vi "RAMP_uptade_scan_steps_indicators.vi"(4 "Total # steps":i32, 5 "error in":errorcluster) -> (6 "slider":u8, 7 "scan step":i32, 8 "error out":errorcluster)   [LabVIEW 2015]
uses:
  GLOBAL/Global_MAIN.vi
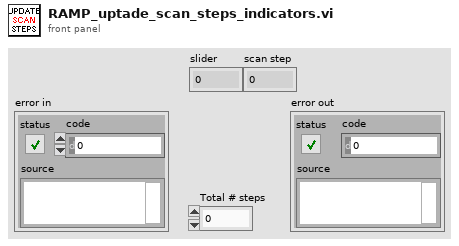
[diagram p1: front panel]
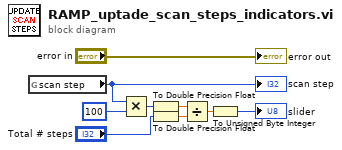
[diagram p0: block diagram]
diagram:
  n1 = global read "Global_MAIN.vi" "scan step"() -> (w6:i32)
  "scan step" <- w6
  n2 = Multiply(x=w6, y=100) -> (x*y=w8:i32)
  n3 = To Double Precision Float(number=w8) -> (double precision float=w2:dbl)
  n4 = To Double Precision Float(number="Total # steps") -> (double precision float=w1:dbl)
  n5 = Divide(x=w2, y=w1) -> (x/y=w7:dbl)
  n6 = To Unsigned Byte Integer(number=w7) -> (unsigned 8bit integer=→"slider":u8)
  "error out" <- "error in"
